vi "Test2_3b_ASIC_mezzanine.vi"(0 "Instrument VISA in":T1={"AWG VISA"="generadorpulsos", "Oscilloscope  VISA "="Oscilloscope", "Integration Board IP"="172.16.7.43", "connection ID"=refnum, "report out"=refnum, "report file path"=path "C:/Documents and Settings/CTA_LAB01/Desktop/L0_Asic/L0 Asic Test Data"}, 5 "quantity":i32=3, 7 "Cycles Burst":i32=10000, 9 "L1 Address":i32=17, 11 "error in":errorcluster, 12 "channel array":i32[](array[numeric])=[0, 1, 2, 3, 4, 5, 6]) -> (4 "Instrument VISA out":T1={"AWG VISA"="", "Oscilloscope  VISA "="", "Integration Board IP"="", "connection ID"=refnum, "report out"=refnum, "report file path"=path "C:/Documents and Settings/CTA_LAB01/Desktop/L0_Asic/L0 Asic Test Data"}, 15 "error out":errorcluster={"status"=TRUE, "code"=63, "source"="TCP Open Connection in Test2_3b_ASIC_mezzanine.vi->test_sum_mezzanine_ASIC.vi"})   [LabVIEW 2009]
uses:
  <vilib>/Utility/NIReport.llb/NI_report.lvclass
  <vilib>/Utility/NIReport.llb/HTML/NI_HTML.lvclass
  <instrlib>/Agilent 81150/Agilent 81150.lvlib
  L0_Asic/L0 Asic Test Folder v9/C/Program Files/National Instruments/LabVIEW 2012/instr.lib/Agilent 8000 Series/Agilent 8000 Series.lvlib
panel:
  out "Filename Out":path
  out "Array":i32[](array[numeric])=[1, 2, 3, 4, 5, 6]
  out "points quantity":dbl=59.0
  out "appended array":dbl[](array[numeric])=[1.0, 126.0, 0.0, 63.0, 3.0, 9.99999e+37, 9.99999e+37, 2.249499e-09, 7.373e-12, 0.44562, 0.00448, 9.99999e+37, 9.99999e+37, 9.99999e+37, 9.99999e+37, 59.0]
  out "read buffer 3":string="V amptd(1),9.99999E+37,9.99999E+37,9.99999E+37,9.99999E+37,9.99999E+37,5.9E+01,+ width(1),2.24799E-09,2.23076E-09,2.26701E-09,2.249499E-09,7.373E-12,5.9E+01,V amptd(f2),4.428E-01,4.360E-01,4.564E-01,4.4562E-01,4.48E-03,5.9E+01,+ width(f2),9.99999E+37,9.99999E+37,9.99999E+37,9.99999E+37,9.99999E+37,9.99999E+37,Time(1-f2),9.99999E+37,9.99999E+37,9.99999E+37,9.99999E+37,9.99999E+37,9.99999E+37\n"
  in  "Quantity of measurements":u32=50
  in  "Voltage":dbl[](array[numeric])=[0.05, 0.2, 0.5, 0.7, 1.0]
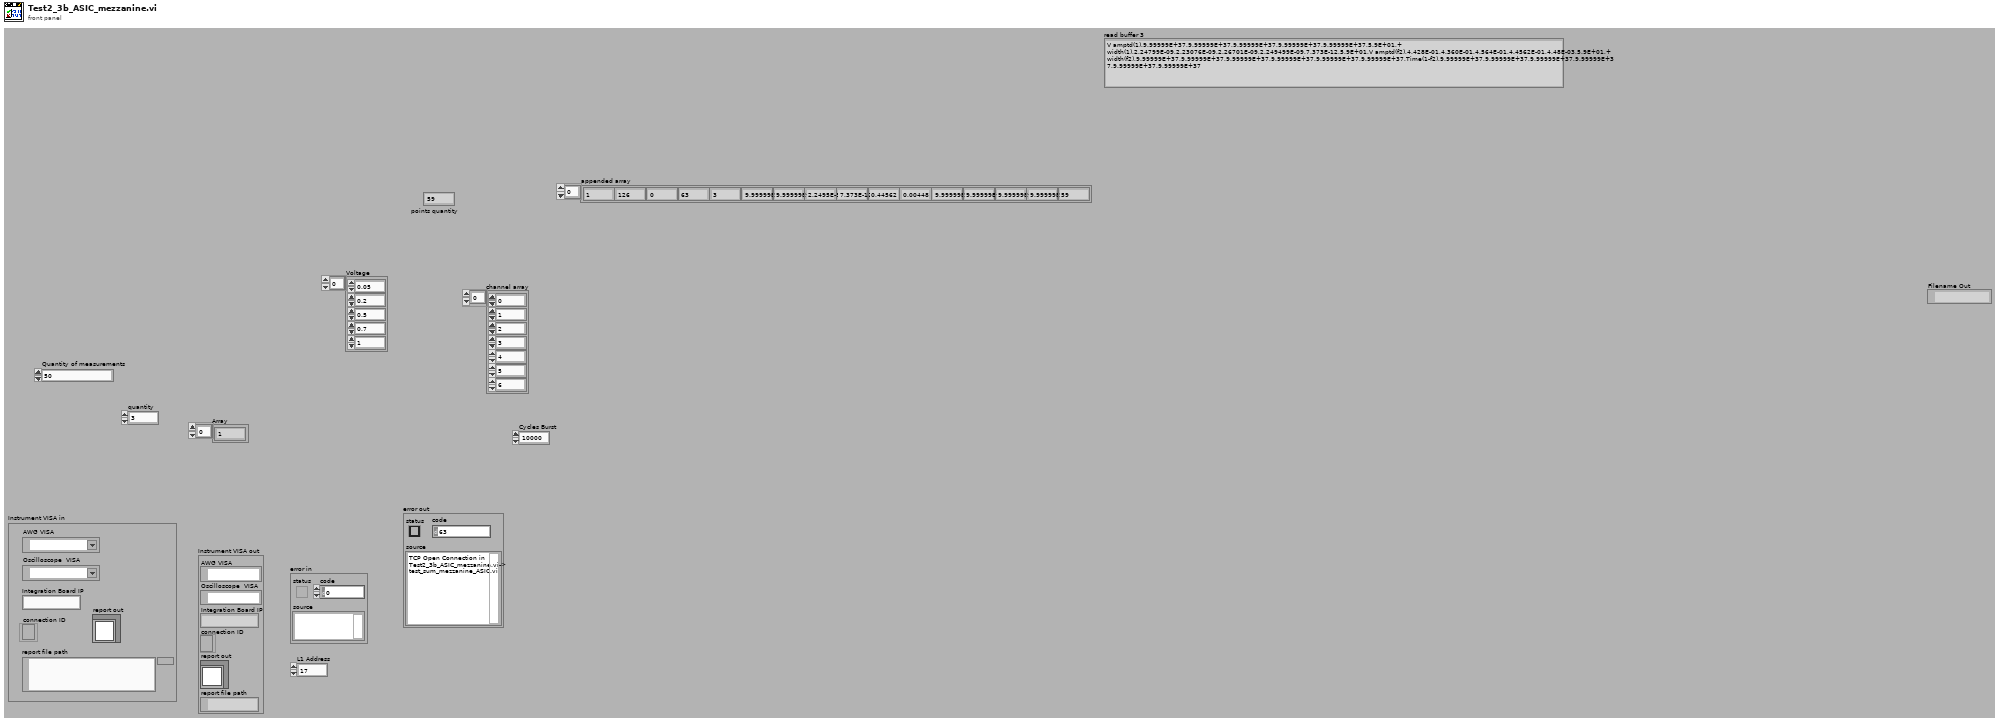
[diagram p1: front panel]
types:
  T1 = cluster{"AWG VISA":refnum<visa-resource-name>, "Oscilloscope  VISA ":refnum<visa-resource-name>, "Integration Board IP":string, "connection ID":refnum<k5>, "report out":refnum<class "NI_report.lvclass">, "report file path":path}
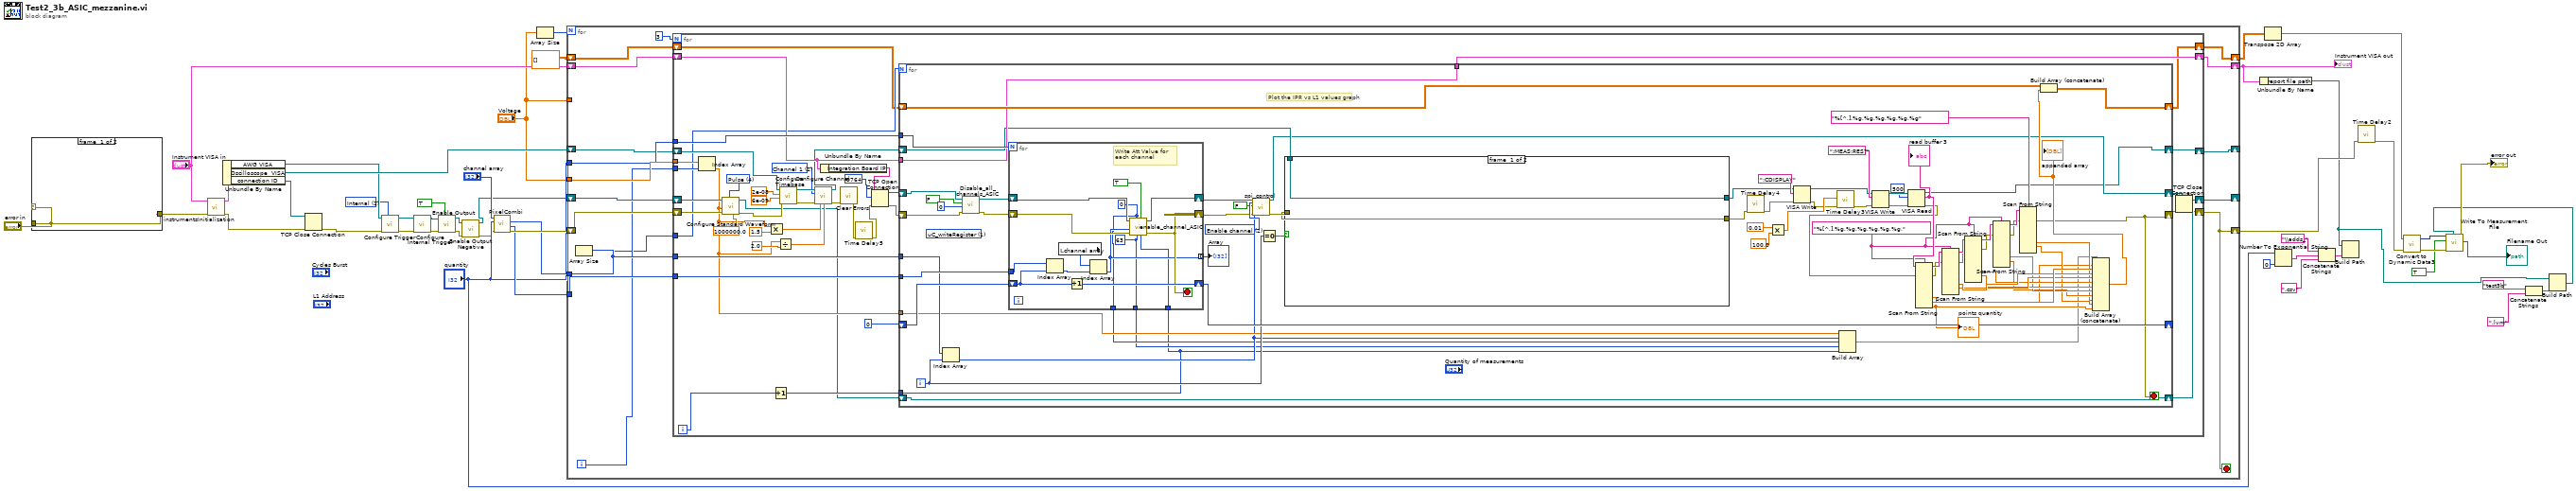
[diagram p0: block diagram]
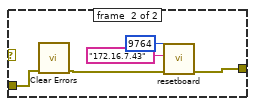
[diagram p2: hidden frame]
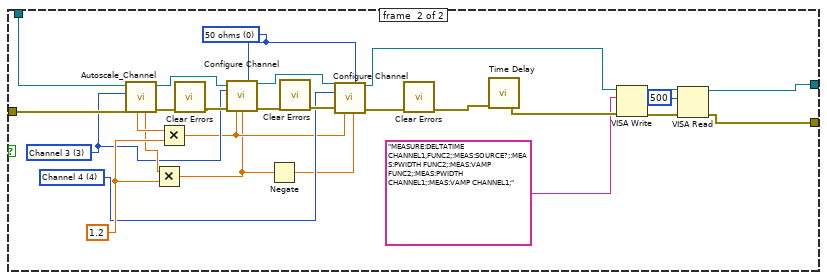
[diagram p3: hidden frame]
diagram:
  w19 = u16 1 items=["Immediate", "Internal", "External", "Software Trigger Function"] ("Trigger Source (0: Immediate)")
  n1 = case shown="Error" "error in" {
    tunnel: "error in" -> [w47 w49]
    tunnel: [w47 w52] -> w15
    frame #0 {
    }
    frame #1 {
      n2 = call <vilib>:"Clear Errors.vi"("error in (no error)"=w49) -> ("error out"=w48:errorcluster)  [unwired: 6 in]
      n3 = call "resetboard.vi"("error in (no error)"=w48, "address"="172.16.7.43", "remote port or service name"=u16 9764) -> ("error out"=w52:errorcluster)  [unwired: 7 in, 1 out]
    }
  }
  n4 = call "instrumentsInitialization.vi"("error in"=w15, "Instrument VISA in"="Instrument VISA in") -> ("error out"=w13:errorcluster, "Instrument VISA out"=w39:T1)  [unwired: 8 in]
  n5 = Unbundle By Name(w39) -> ("AWG VISA"=w22:refnum<visa-resource-name>, "Oscilloscope  VISA"=w38:refnum<visa-resource-name>, "connection ID"=w14:refnum<k5>)
  n6 = TCP Close Connection(connection ID=w14, error in (no error)=w13) -> (error out=w12:errorcluster)  [unwired: 1 in, 1 out]
  n7 = call <instrlib>:"Configure Trigger.vi"("Trigger Source (0: Immediate)"=w19, "error in (no error)"=w12, "VISA resource name"=w22) -> ("error out"=w20:errorcluster, "VISA resource name out"=w21:refnum<visa-resource-name>)  [unwired: 7 in]
  n8 = call <instrlib>:"Configure Internal Trigger.vi"("error in (no error)"=w20, "VISA resource name"=w21) -> ("error out"=w23:errorcluster, "VISA resource name out"=w24:refnum<visa-resource-name>)  [unwired: 8 in]
  n9 = call <instrlib>:"Enable Output.vi"("Enable Output (T: Enable)"=TRUE, "error in (no error)"=w23, "VISA resource name"=w24) -> ("error out"=w9:errorcluster, "VISA resource name out"=w8:refnum<visa-resource-name>)  [unwired: 7 in]
  n10 = call <instrlib>:"Enable Output Negative.vi"("error in (no error)"=w9, "VISA resource name"=w8) -> ("error out"=w10:errorcluster, "VISA resource name out"=w11:refnum<visa-resource-name>)  [unwired: 8 in]
  n11 = call "PixelCombi.vi"("error in"=w10, "quantity"="quantity", "array"="channel array") -> ("error out"=w45:errorcluster, "Channels"=w44:i32[], "Combination Array"=w43:i16[])  [unwired: 6 in]
  n12 = Array Size(array="Voltage") -> (size(s)=w40:i32)
  n13 = for {
    N: w40 -> [_]
    tunnel: w44 -> [w67]
    tunnel: w43 -> [w66]
    shift-right: [w53] -> w26
    shift-left: w45 -> [w69]
    tunnel: "Voltage" -> [w65]
    tunnel: "Voltage" -> [_]
    tunnel: "quantity" -> [w63]
    shift-right: [w58] -> w25
    shift-left: "Instrument VISA in" -> [w61]
    shift-right: [w57] -> w29
    shift-left: dbl[][] [] -> [w59]
    shift-right: [w54] -> _
    shift-left: w11 -> [w68]
    shift-right: [w55] -> _
    shift-left: w38 -> [w62]
    i -> [w64]
    stop <- w53 stop-if-true
    n14 = Array Size(array=w66) -> (size(s)=w60:i32)
    n15 = for {
      N: 3 -> [_]
      tunnel: w67 -> [w108]
      tunnel: w66 -> [w106]
      tunnel: w65 -> [w105]
      tunnel: w64 -> [w104]
      tunnel: w63 -> [w103]
      tunnel: w60 -> [w88]
      shift-right: [w78] -> w57
      shift-left: w59 -> [w81]
      shift-right: [w79] -> w58
      shift-left: w61 -> [w92]
      shift-right: [w73] -> w53
      shift-left: w69 -> [w110]
      shift-right: [w74] -> w54
      shift-left: w68 -> [w109]
      shift-right: [w76] -> w55
      shift-left: w62 -> [w99]
      i -> [w70]
      w95 = 1 items=["Channel 1"=1, "Channel 2"=2, "Channel 3"=3, "Channel 4"=4] ("Channel (1: Channel 1)")
      w112 = u16 4 items=["Sine", "Square", "Ramp Up", "Ramp Down", "Pulse", "Noise", "DC"] ("Waveform (0: Sine)")
      n16 = Index Array(array=w105, index=w104) -> (element=w80:dbl)
      n17 = call <instrlib>:"Configure Standard Waveform.vi"("Frequency (1000.0 Hz)"=1000000.0, "Waveform (0: Sine)"=w112, "error in (no error)"=w110, "Amplitude (1.0 Vpp)"=w80, "VISA resource name"=w109) -> ("error out"=w102:errorcluster, "VISA resource name out"=w75:refnum<visa-resource-name>)  [unwired: 5 in]
      n18 = Multiply(x=w80, y=1.5) -> (x*y=w94:dbl)
      n19 = Increment(x=w70) -> (x+1=w77:i32)
      n20 = Divide(x=w80, y=2.0) -> (x/y=w86:dbl)
      n21 = call <instrlib>:"Configure Timebase.vi"("error in (no error)"=w102, "Position (0.0 s)"=6e-09, "Timebase (0.005 s)"=2e-08, "VISA resource name"=w99) -> ("error out"=w101:errorcluster, "VISA resource name out"=w98:refnum<visa-resource-name>)  [unwired: 6 in]
      n22 = call <instrlib>:"Configure Channel.vi"("VISA resource name"=w98, "Channel (1: Channel 1)"=w95, "error in (no error)"=w101, "Vertical Range (2.0 V)"=w94, "Vertical Offset (0.0 V)"=w86) -> ("VISA resource name out"=w85:refnum<visa-resource-name>, "error out"=w100:errorcluster)  [unwired: 9 in]
      n23 = Unbundle By Name(w92) -> ("Integration Board IP"=w90:string)
      n24 = call <vilib>:"Clear Errors.vi"("error in (no error)"=w100) -> ("error out"=w72:errorcluster)  [unwired: 6 in]
      n25 = call "Time Delay5"("error in (no error)"=w72) -> ("error out"=w71:errorcluster)  [unwired: 10 in]
      n26 = TCP Open Connection(address=w90, remote port or service name=u16 9764, error in (no error)=w71) -> (connection ID=w82:refnum<k5>, error out=w91:errorcluster)  [unwired: 2 in]
      n27 = for {
        N: w88 -> [_]
        tunnel: w106 -> [w180]
        tunnel: w108 -> [w181]
        shift-right: [w182] -> _
        shift-left: i16 0 ("element") -> [w183]
        shift-right: [w127] -> w84
        shift-left: w91 -> [w173]
        tunnel: w92 -> [w168]
        tunnel: w103 -> [w179]
        tunnel: [w168] -> w79
        shift-right: [w174] -> w78
        shift-left: w81 -> [w175]
        shift-right: [w128] -> w83
        shift-left: w82 -> [w126]
        tunnel: w80 -> [w123]
        tunnel: w77 -> [w118]
        shift-right: [w117] -> w76
        shift-left: w85 -> [w166]
        shift-right: [w116] -> w74
        shift-left: w75 -> [w116]
        i -> [w164]
        stop <- w127 stop-if-true
        w149 = "%[^,],%g,%g,%g,%g,%g,%g," ("format string")
        w172 = u16 2 items=["Attenuation", "Clipping", "Enable channel", "Delay line", "ASIC"] ("Device")
        (unwired) u16 1 items=["sendCommand"=9, "FPGA_writeRegister"=3, "FPGA_readRegister"=2, "uC_writeRegister"=1, "uC_readRegister"=0] ("Action")
        # "Plot the IPR vs L1 values graph"
        n28 = Index Array(array=w180, index=w164) -> (element=w122:i16)
        n29 = call "Disable_all_channels_ASIC.vi"("error in"=w173, "id_in"=0 ("Data"), "Clip_en_b"=FALSE, "connection ID"=w126) -> ("error out"=w177:errorcluster, "connection ID out"=w176:refnum<k5>)  [unwired: 5 in, 1 out]
        n30 = for {
          N: w179 -> [_]
          shift-right: [w225] -> w182
          shift-left: w183 -> [w226]
          tunnel: w181 -> [w224]
          shift-right: [w221] -> w170
          shift-left: w177 -> [w220]
          shift-right: [w218] -> w169
          shift-left: w176 -> [w219]
          tunnel: [w217] -> w125 mode=indexing
          tunnel: [w216] -> w121
          tunnel: [w215] -> w120
          tunnel: w118 -> [w214]
          stop <- w221 stop-if-true
          w216 = u32 0 ("Att gain")
          w215 = u32 63 ("Ib_clipVb")
          # "Write Att Value for each channel"
          n31 = Index Array(array=w224, index=w226) -> (element=w222:i32)
          n32 = local read "channel array"() -> (w223:i32[])
          n33 = Increment(x=w226) -> (x+1=w225:i16)
          n34 = Index Array(array=w223, index=w222) -> (element=w217:i32)
          n35 = call "enable_channel_ASIC.vi"("Clip_sel_b"=w214, "maj/sum"=TRUE, "Ib_clipVb"=w215, "Att gain"=w216, "error in"=w220, "Channel"=w217, "connection ID"=w219) -> ("error out"=w221:errorcluster, "connection ID out"=w218:refnum<k5>)  [unwired: 2 in, 1 out]
        }
        "Array" <- w125
        n36 = call "spi_control.vi"("connection ID"=w169, "Device"=w172, "Read/#write"=FALSE, "Data"=w122, "error out 3"=w170) -> ("connection ID out"=w128:refnum<k5>, "error out 2"=w167:errorcluster)  [unwired: 7 in, 6 out]
        n37 = Equal To 0?(x=w164) -> (x = 0?=w165:bool)
        n38 = case shown="True" w165 {
          tunnel: [w185 w192] -> w113
          tunnel: w167 -> [w185 w198]
          tunnel: w166 -> [w184 w199]
          tunnel: [w184 w201] -> w131
          frame #0 {
          }
          frame #1 {
            w202 = u32 0 items=["50 ohms", "1 Mohms"] ("Input Impedance (1: 1 Mohms)")
            w190 = 3 items=["Channel 1"=1, "Channel 2"=2, "Channel 3"=3, "Channel 4"=4] ("Channel (1: Channel 1)")
            w189 = 4 items=["Channel 1"=1, "Channel 2"=2, "Channel 3"=3, "Channel 4"=4] ("Channel (1: Channel 1)")
            w195 = 1.2 ("y")
            n39 = call "Autoscale_Channel.vi"("error in"=w198, "Channel"=w190, "VISA resource name"=w199) -> ("error out"=w209:errorcluster, "VISA resource name out"=w212:refnum<visa-resource-name>, "Offset"=w191:dbl, "VerticalRange"=w206:dbl)  [unwired: 5 in]
            n40 = Multiply(x=w191, y=w195) -> (x*y=w187:dbl)
            n41 = Multiply(x=w206, y=w195) -> (x*y=w188:dbl)
            n42 = call <vilib>:"Clear Errors.vi"("error in (no error)"=w209) -> ("error out"=w210:errorcluster)  [unwired: 6 in]
            n43 = call <instrlib>:"Configure Channel.vi"("VISA resource name"=w212, "Input Impedance (1: 1 Mohms)"=w202, "Channel (1: Channel 1)"=w190, "error in (no error)"=w210, "Vertical Range (2.0 V)"=w188, "Vertical Offset (0.0 V)"=w187) -> ("VISA resource name out"=w207:refnum<visa-resource-name>, "error out"=w211:errorcluster)  [unwired: 8 in]
            n44 = Negate(x=w187) -> (-x=w186:dbl)
            n45 = call <vilib>:"Clear Errors.vi"("error in (no error)"=w211) -> ("error out"=w200:errorcluster)  [unwired: 6 in]
            n46 = call <instrlib>:"Configure Channel.vi"("VISA resource name"=w207, "Input Impedance (1: 1 Mohms)"=w202, "Channel (1: Channel 1)"=w189, "error in (no error)"=w200, "Vertical Range (2.0 V)"=w188, "Vertical Offset (0.0 V)"=w186) -> ("VISA resource name out"=w196:refnum<visa-resource-name>, "error out"=w208:errorcluster)  [unwired: 8 in]
            n47 = call <vilib>:"Clear Errors.vi"("error in (no error)"=w208) -> ("error out"=w197:errorcluster)  [unwired: 6 in]
            n48 = call "Time Delay"("error in (no error)"=w197) -> ("error out"=w194:errorcluster)  [unwired: 10 in]
            n49 = VISA Write(VISA resource name=w196, write buffer="MEASURE:DELTATIME CHANNEL1,FUNC2;:MEAS:SOURCE?;:MEAS:PWIDTH FUNC2;:MEAS:VAMP FUNC2;:MEAS:PWIDTH CHANNEL1;:MEAS:VAMP CHANNEL1;", error in (no error)=w194) -> (VISA resource name out=w205:refnum<visa-resource-name>, error out=w204:errorcluster)  [unwired: 1 out]
            n50 = VISA Read(VISA resource name=w205, byte count=u32 500, error in (no error)=w204) -> (VISA resource name out=w201:refnum<visa-resource-name>, error out=w192:errorcluster)  [unwired: 2 out]
          }
        }
        n51 = call "Time Delay4"("error in (no error)"=w113) -> ("error out"=w114:errorcluster)  [unwired: 10 in]
        n52 = Multiply(x=0.01, y=100.0) -> (x*y=w156:dbl)
        n53 = VISA Write(VISA resource name=w131, write buffer=":CDISPLAY", error in (no error)=w114) -> (VISA resource name out=w134:refnum<visa-resource-name>, error out=w132:errorcluster)  [unwired: 1 out]
        n54 = call "Time Delay3"("error in (no error)"=w132, "Delay Time (s)"=w156) -> ("error out"=w155:errorcluster)  [unwired: 9 in]
        n55 = Build Array(w123, w122, w121, w120, w118) -> (w119:dbl[])
        n56 = VISA Write(VISA resource name=w134, write buffer=":MEAS:RES?", error in (no error)=w155) -> (VISA resource name out=w163:refnum<visa-resource-name>, error out=w162:errorcluster)  [unwired: 1 out]
        n57 = VISA Read(VISA resource name=w163, byte count=u32 500, error in (no error)=w162) -> (VISA resource name out=w117:refnum<visa-resource-name>, read buffer=w159:string, error out=w139:errorcluster)  [unwired: 1 out]
        "read buffer 3" <- w159
        n58 = Scan From String(format string=w149, input string=w159, error in=w139) -> (remaining string=w153:string, error out=w135:errorcluster, output 5=w124:dbl, output 6=w154:dbl, output 7=w140:dbl)  [unwired: 12 in, 1 out]
        "points quantity" <- w140
        n59 = Scan From String(format string=w149, input string=w153, error in=w135) -> (remaining string=w150:string, error out=w136:errorcluster, output 5=w147:dbl, output 6=w146:dbl)  [unwired: 13 in, 1 out]
        n60 = Scan From String(format string=w149, input string=w150, error in=w136) -> (remaining string=w151:string, error out=w137:errorcluster, output 5=w145:dbl, output 6=w144:dbl)  [unwired: 13 in, 1 out]
        n61 = Scan From String(format string=w149, input string=w151, error in=w137) -> (remaining string=w152:string, error out=w138:errorcluster, output 5=w143:dbl, output 6=w142:dbl)  [unwired: 13 in, 1 out]
        n62 = Scan From String(format string="%[^,],%g,%g,%g,%g,%g,%g", input string=w152, error in=w138) -> (error out=w127:errorcluster, output 5=w130:dbl, output 6=w141:dbl)  [unwired: 13 in, 2 out]
        n63 = Build Array (concatenate)(w119, w124, w154, w147, w146, w145, w144, w143, w142, w130, w141, w140) -> (w129:dbl[])
        "appended array" <- w129
        n64 = Build Array (concatenate)(w175, w129) -> (w174:dbl[][])
      }
      n65 = TCP Close Connection(connection ID=w83, error in (no error)=w84) -> (error out=w73:errorcluster)  [unwired: 1 in, 1 out]
    }
  }
  "Instrument VISA out" <- w25
  n66 = Unbundle By Name(w25) -> ("report file path"=w1:path)
  n67 = Transpose 2D Array(2D array=w29) -> (transposed array=w17:dbl[][])
  n68 = Number To Exponential String(number="quantity", precision (6)=i16 0) -> (E-format string=w33:string)  [unwired: 2 in]
  n69 = Concatenate Strings("\\adds_" ("string"), w33, ".csv" ("name or relative path")) -> (w36:string)
  n70 = Build Path(base path=w1, name or relative path=w36) -> ()  [unwired: 1 out]
  n71 = call "Time Delay2"("error in (no error)"=w26) -> ("error out"=w41:errorcluster)  [unwired: 10 in]
  n72 = call "Convert to Dynamic Data3"("2D Array"=w17) -> ("Dynamic Data Type"=w18:dynamicdata)  [unwired: 3 in]
  n73 = Concatenate Strings("test3b" ("string"), ".lvm" ("name or relative path")) -> (w7:string)
  n74 = Build Path(base path=w1, name or relative path=w7) -> (appended path=w3:path)
  n75 = call "Write To Measurement File"("Signals"=w18, "Enable"=TRUE, "error in (no error)"=w41, "Filename"=w3) -> ("Filename Out"=→"Filename Out":path, "error out"=→"error out":errorcluster)  [unwired: 13 in, 1 out]
